vi "Global.vi"() -> ()   [LabVIEW 2021, in "Markdown.lvlib"]
doc: "Markdown global variables. This library uses a global variable to avoid large data flow copies."
uses:
  Markdown.lvlib
  TypeDefs/Item.ctl
panel:
  in  "VI ConPane Images":path[](array[path])
  in  "VI ConPane Idxs":i32[](array[numeric])
  in  "VI Tree Idxs":i32[](array[numeric])
  in  "Palette Names":string[](array[string])
  in  "Palette Images":path[](array[path])
  in  "Ex Idxs":i32[](array[numeric])
  in  "Ex Images":path[](array[path])
  in  "Items":T1[](array[typedef])
  in  "Item Refnums":refnum<vi>[](array[refnum])
  in  "Summary":string
  in  "Library Refnum":refnum<vi>
  in  "Library.lvlib":path
  in  "API.md":path
  in  "ImgDir":path
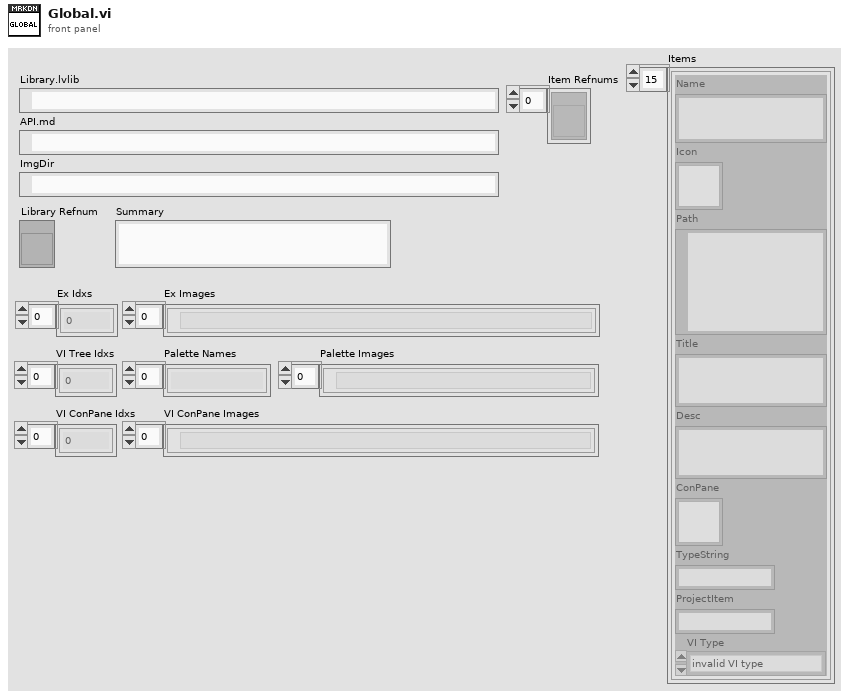
[diagram p1: front panel]
types:
  T1 = typedef "Markdown.lvlib/Item.ctl" = cluster{"Name":string, "Icon":picture, "Path":path, "Title":string, "Desc":string, "ConPane":picture, "TypeString":string, "ProjectItem":string, "VI Type":enum32{"invalid VI type", "Standard VI", "Control VI", "Global VI", "Polymorphic VI", "Configuration VI", "SubSystem", "Facade VI", "Method VI", "Statechart Diagram VI"}}
diagram:
